vi "udp rx.vi"() -> ()   [LabVIEW 2019]
panel:
  out "appended array":bool[](array[boolean])
  in  "receiver port":u16=8089
  out "data out":string
  in  "Stop":bool
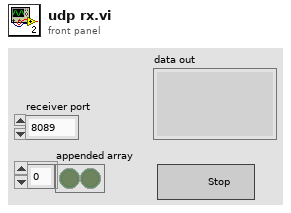
[diagram p1: front panel]
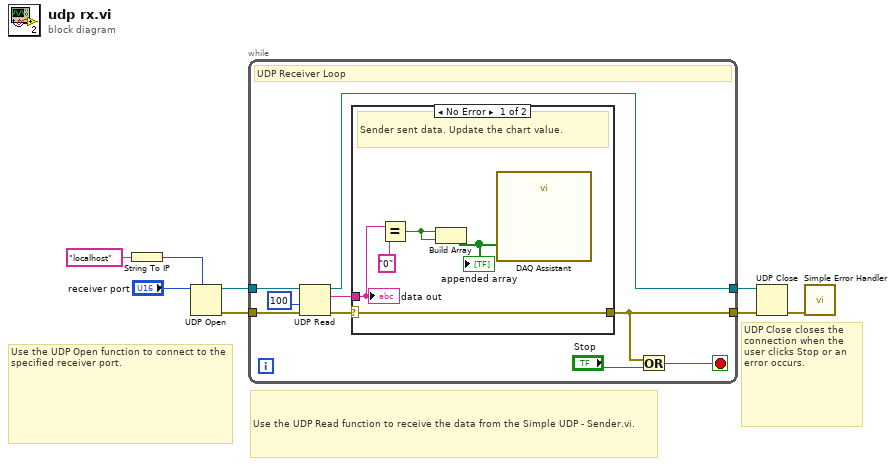
[diagram p0: block diagram]
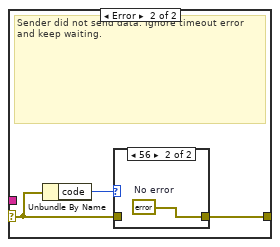
[diagram p2: hidden frame]
diagram:
  # "UDP Close closes the connection when the user clicks Stop or an error occurs."
  # "Use the UDP Open function to connect to the specified receiver port."
  # "Use the UDP Read function to receive the data from the Simple UDP - Sender.vi."
  n1 = String To IP(1:"localhost" ("name")) -> (0:w1:u32)
  n2 = UDP Open(7:w1, 11:"receiver port") -> (port=w4:refnum<k16>, 0:w5:errorcluster)  [unwired: 3 in, 1 out]
  n3 = while {
    tunnel: w4 -> [w17]
    tunnel: [w9] -> w8
    tunnel: w5 -> [w14]
    tunnel: [w10] -> w6
    stop <- w15 stop-if-true
    # "UDP Receiver Loop"
    n4 = UDP Read(connection ID=w17, timeout ms (25000)=100, 8:w14) -> (data out=w12:string, error out=w11:errorcluster, 3:w9:refnum<k16>)  [unwired: 3 out]
    n5 = case shown="No Error" w11 {
      selector: w11 -> [w22 w24]
      tunnel: w12 -> [w21 _]
      tunnel: [w22 w23] -> w10
      frame No Error {
        # "Sender sent data. Update the chart value."
        n6 = Equal?(x=w21, y="0") -> (x = y?=w19:bool)
        n7 = Build Array(w19, w19) -> (w18:bool[])
        "appended array" <- w18
        n8 = call "DAQ Assistant"("data"=w18) -> ()  [unwired: 17 in, 2 out]
        "data out" <- w21
      }
      frame Error {
        # "Sender did not send data. Ignore timeout error and keep waiting."
        n9 = Unbundle By Name(w24) -> ("code"=w25:i32)
        n10 = case shown="56" w25 {
          tunnel: w24 -> [w26 _]
          tunnel: [w26 w27] -> w23
          frame Default {
          }
          frame 56 {
            w27 = errorcluster {"status"=FALSE, "code"=0, "source"=""}  # No error
          }
        }
      }
    }
    n11 = Or(x=w10, y="Stop") -> (x .or. y?=w15:bool)
  }
  n12 = UDP Close(connection ID=w8, 8:w6) -> (error out=w7:errorcluster)  [unwired: 1 out]
  n13 = call <vilib>:"Simple Error Handler.vi"("error in (no error)"=w7) -> ()  [unwired: 1 in, 8 out]
